vi "aft_xmpl_Simulate Expected Waveform (FXP).vi"(11 "Amplitude":dbl) -> (3 "signal":i32[](array[numeric]))   [LabVIEW 2023]
uses:
  <vilib>/Analysis/3filter.llb/Butterworth Filter (DBL).vi
  <vilib>/Analysis/NI_AALBase.lvlib
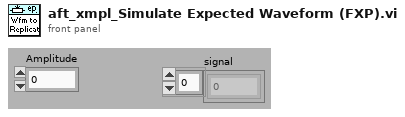
[diagram p1: front panel]
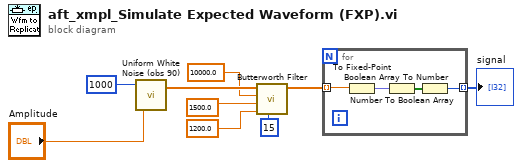
[diagram p0: block diagram]
diagram:
  n1 = call <vilib>:"Uniform White Noise (obs 90).vi"("amplitude"="Amplitude", "samples"=1000) -> ("uniform white noise"=w8:dbl[])  [unwired: 1 in, 1 out]
  n2 = call-poly <vilib>:"Butterworth Filter.vi"("order"=15, "low cutoff freq: fl"=1200.0, "high cutoff freq: fh"=1500.0, "sampling freq: fs"=10000.0 ("y"), "X"=w8) -> ("Filtered X"=w9:dbl[])  [unwired: 2 in, 2 out]
  n3 = for {
    tunnel: w9 -> [w13] mode=indexing
    tunnel: [w10] -> w1 mode=indexing
    n4 = To Fixed-Point(number=w13) -> (fixed-point=w12:fxp<+/-,24,4>)  [unwired: 1 out]
    n5 = Number To Boolean Array(number=w12) -> (Boolean array=w11:bool[])
    n6 = Boolean Array To Number(Boolean array=w11) -> (number=w10:i32)
  }
  "signal" <- w1
